vi "piezoDoubleSimple.vi"() -> ()   [LabVIEW 2017]
panel:
  in  "piezo1 0":dbl=100.0 format="%#_13g"
  in  "coef 3":dbl format="%04.6f"
  in  "coef 2":dbl=0.0015000000000000002 format="%04.6f"
  in  "piezo2 0":dbl=100.0 format="%.2f"
  in  "calc":bool
  in  "piezo 2":dbl=100.0 min=0.0 max=200.0 step=0.5 format="%1.2f"
  in  "coef":dbl=-0.5 format="%04.4f"
  in  "stop":bool
  out "piezo2 set":dbl
  in  "piezo1":dbl=100.0 min=0.0 max=200.0 format="%.2g"
  # "0.001500"
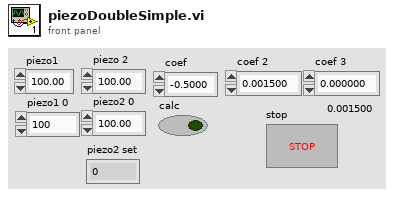
[diagram p1: front panel]
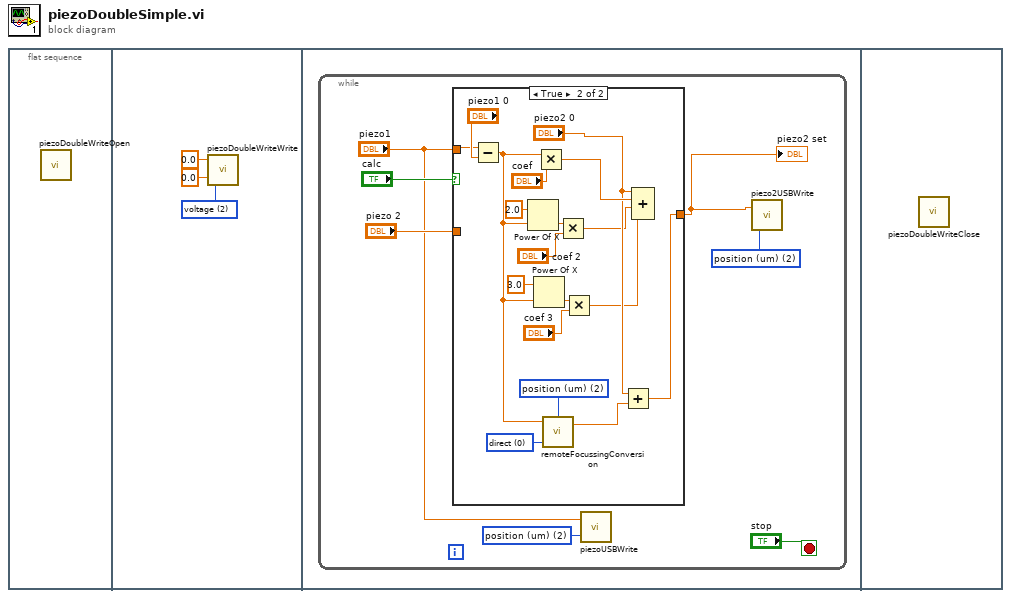
[diagram p0: block diagram]
diagram:
  n1 = flat-sequence {
    frame #0 {
      n2 = call "piezoDoubleWriteOpen.vi"() -> ()  [unwired: 2 in]
    }
    frame #1 {
      w1 = u16 2 items=["fractional", "position", "voltage"] ("mode")
      n3 = call "piezoDoubleWriteWrite.vi"("mode"=w1, "piezo2"=0.0, "piezo1"=0.0) -> ()  [unwired: 1 in]
    }
    frame #2 {
      n4 = while {
        stop <- "stop" stop-if-true
        w4 = u16 2 items=["fractional", "voltage (V)", "position (um)"] ("mode")
        w6 = u16 2 items=["fractional", "voltage (V)", "position (um)"] ("mode")
        n5 = case shown="True" "calc" {
          tunnel: "piezo1" -> [_ w26]
          tunnel: [w11 w12] -> w7
          tunnel: "piezo 2" -> [w11 _]
          frame False {
          }
          frame True {
            w13 = u16 2 items=["fractional", "voltage (V)", "position (um)"] ("units")
            w25 = u16 0 items=["direct", "inverse"] ("mode")
            n6 = Subtract(x=w26, y="piezo1 0") -> (x-y=w19:dbl)
            n7 = Power Of X(1:w19, 2:2.0 ("y")) -> (0:w23:dbl)
            n8 = Power Of X(1:w19, 2:3.0 ("y")) -> (0:w21:dbl)
            n9 = Multiply(x=w19, y="coef") -> (x*y=w17:dbl)
            n10 = call "remoteFocussingConversion.vi"("units"=w13, "mode"=w25, "dz"=w19) -> ("dz out"=w24:dbl)  [unwired: 1 in, 1 out]
            n11 = Multiply(x=w23, y="coef 2") -> (x*y=w15:dbl)
            n12 = Multiply(x=w21, y="coef 3") -> (x*y=w14:dbl)
            n13 = Add(x="piezo2 0", y=w24) -> (x+y=w12:dbl)
            n14 = Compound Arithmetic op=ADD("piezo2 0", w17, w15, w14) -> ()  [unwired: 1 out]
          }
        }
        "piezo2 set" <- w7
        n15 = call "piezoUSBWrite.vi"("mode"=w4, "position"="piezo1") -> ()  [unwired: 1 in]
        n16 = call "piezo2USBWrite.vi"("mode"=w6, "position"=w7) -> ()  [unwired: 1 in]
      }
    }
    frame #3 {
      n17 = call "piezoDoubleWriteClose.vi"() -> ()  [unwired: 1 in]
    }
  }
